vi "case struct.vi"() -> ()   [LabVIEW 2020]
uses:
  <vilib>/ErrorRing/Error Ring.xnode
panel:
  in  "String":string
  in  "Numeric":u16
  in  "Boolean":bool
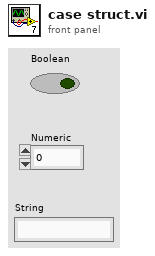
[diagram p1: front panel]
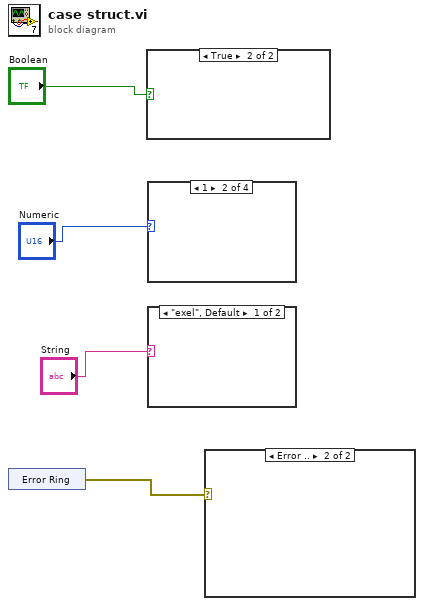
[diagram p0: block diagram]
diagram:
  n1 = xnode "Error Ring"() -> ("error out"=w1:errorcluster)
  n2 = case shown="True" "Boolean" {
    frame False {
    }
    frame True {
    }
  }
  n3 = case shown="1" "Numeric" {
    frame 0, Default {
    }
    frame 1 {
    }
    frame 2 {
    }
    frame 3 {
    }
  }
  n4 = case shown="\"exel\", Default" "String" {
    frame "exel", Default {
    }
    frame "a" {
    }
  }
  n5 = case shown="Error .." w1 {
    frame No Error {
    }
    frame Error {
    }
  }
